vi "VESASignal_Run.vi"   [LabVIEW 2020]
uses:
  <vilib>/Platform/TimedLoop/XDataNode/timing_clust.ctl
  <vilib>/Platform/TimedLoop/XDataNode/nitl_modes.ctl
  <vilib>/Platform/TimedLoop/XDataNode/wakeup.ctl
  <vilib>/rvi/Emulation/niFpgaSctlEmulationGetInTimedLoop.vi
  <vilib>/rvi/Emulation/niFpgaEmulationReportErrorSimple.vi
  <vilib>/rvi/Emulation/niFpgaGetClockAttributes.vi
  <vilib>/rvi/Emulation/niFpgaCriticalErrorInLSC.vi
  <vilib>/rvi/Memory/Memory_Emulation/nirvimemoryFastEmulation.vi
  <vilib>/rvi/Memory/Memory_Emulation/nirvimemoryEmulation.vi
  <vilib>/rvi/Emulation/niFpgaEmulationIsFPGAContextNoSignature.vi
  <vilib>/rvi/DataTransferAndStorage/Container/Common/niFpgaContainerGetUniqueNameForEmu.vi
  <vilib>/rvi/Emulation/niFpgaProcessEmulError.vi
  <vilib>/rvi/errors/nirviReportUnexpectedCaseInternalError (U32).vi
  <vilib>/rvi/eio/common/nirviEmuTemplateMethod_errors.vi
  <vilib>/Platform/TimedLoop/XDataNode/XDataNode.xnode
  <vilib>/rvi/DataTransferAndStorage/Container/XNode/niFpgaContainer.xnode
  <vilib>/eio/EIONode/EIONode.xnode
  <vilib>/Platform/TimedLoop/XDataNode/XDNodeRunTimeDep.lvlib
types:
  T1 = typedef "XDNodeRunTimeDep.lvlib/timing_clust.ctl" = cluster{"Expected End [f-1]":u64, "Actual End [f-1]":u64, "Finished Late? [f-1]":bool, "Expected End [i-1]":u64, "Actual End [i-1]":u64, "Finished Late? [i-1]":bool, "Expected Start [i]":u64, "Actual Start [i]":u64, "Expected Start [f]":u64, "Actual Start [f]":u64, "Source Name":string, "Structure Name":string, "Period":i64, "Deadline":i64, "Offset":i64, "Start":i64, "Priority":i32, "Timeout":i32, "Mode":T2, "Wakeup Reason":T3, "Error":errorcluster, "Source Type":string, "Secondary Source Type":string, "Global End Time":u64, "Global Start Time":u64, "Frame Duration":u64, "Iteration Duration":u64, "Assigned CPU":i32, "I/O Scan Engine Mode":u32}
  T2 = typedef "XDNodeRunTimeDep.lvlib/nitl_modes.ctl" = enum32{"No Change", "Process missed periods, maintain original phase", "Discard missed periods, maintain original phase", "Process missed periods, ignore original phase", "Discard missed periods, ignore original phase"}
  T3 = typedef "XDNodeRunTimeDep.lvlib/wakeup.ctl" = enum32{"Normal", "Aborted", "Asynchronous wakeup", "Timing source error", "Timed loop error", "Timeout"}
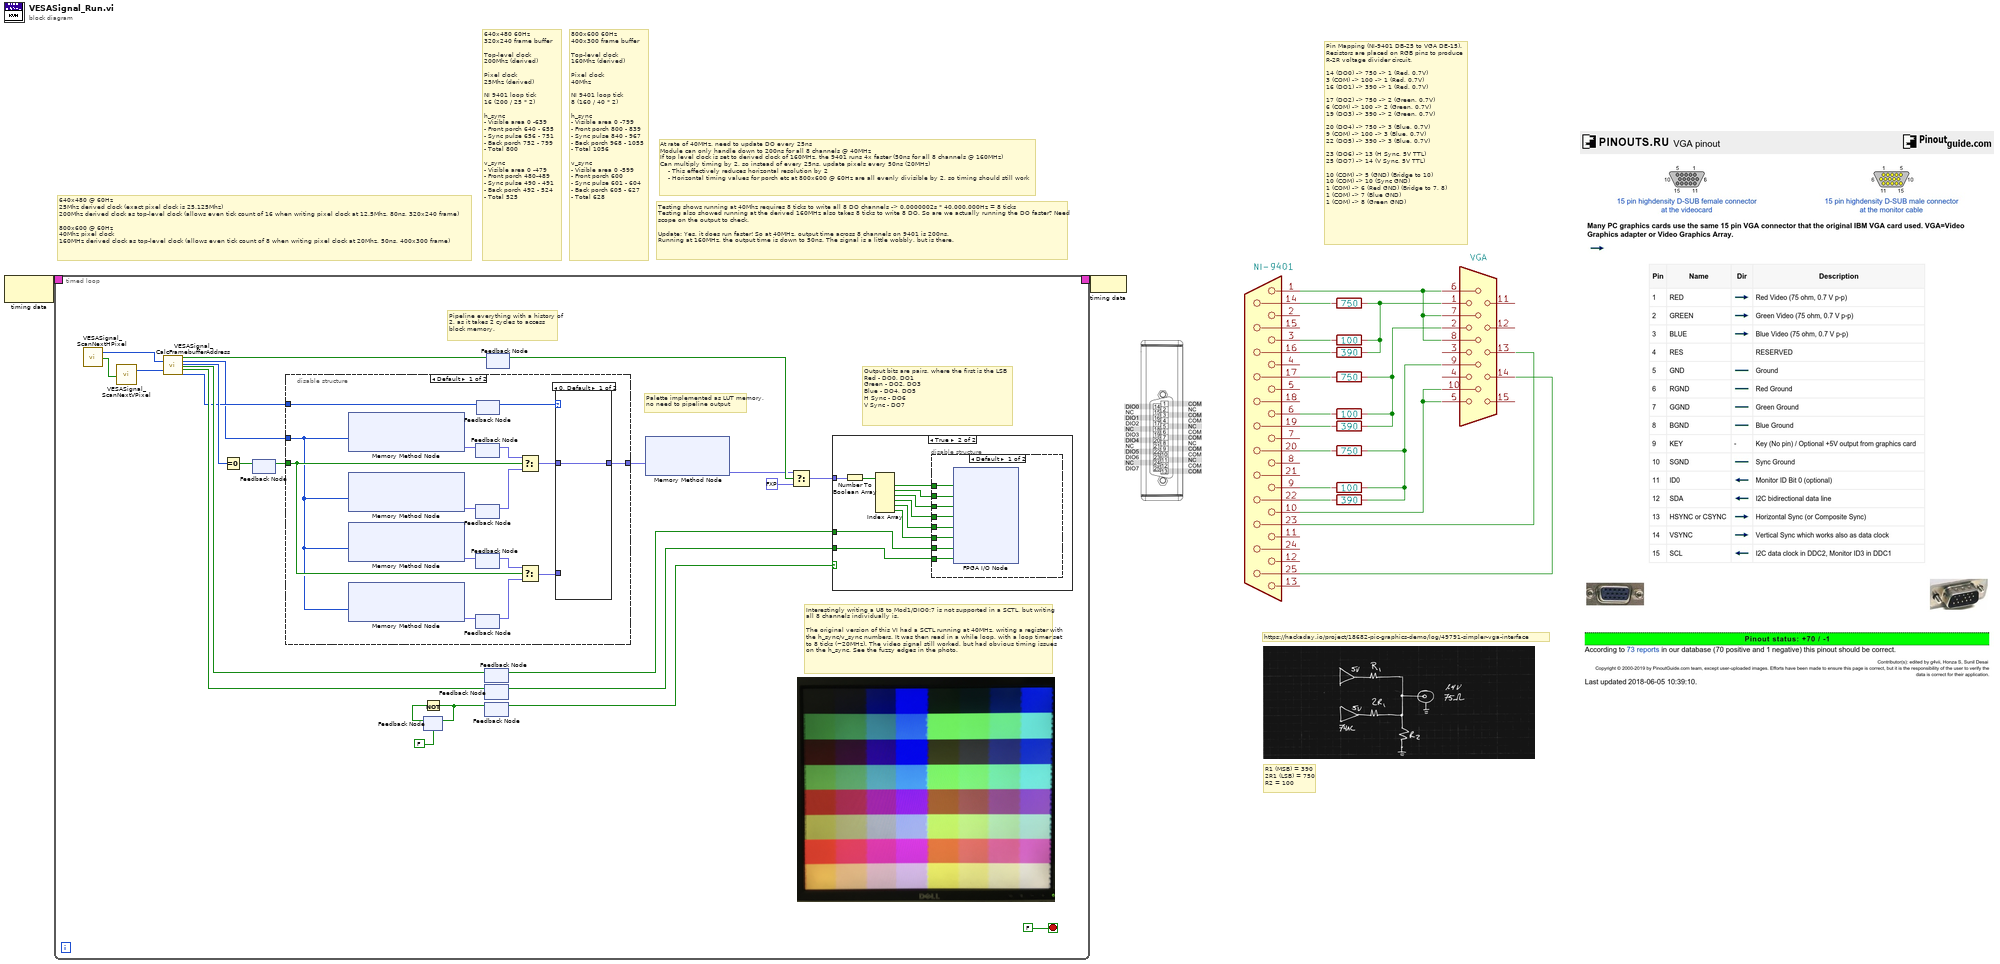
[diagram p0: block diagram]
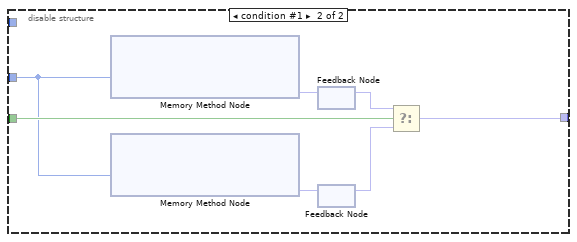
[diagram p3: hidden frame]
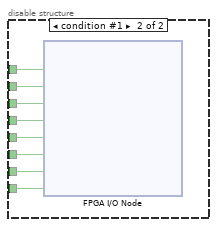
[diagram p5: hidden frame]
diagram:
  # "https://hackaday.io/project/18682-pic-graphics-demo/log/49791-simpler-vga-interface"
  # "R1 (MSB) = 390\n2R1 (LSB) = 750\nR2 = 100"
  # "Pin Mapping (NI-9401 DB-25 to VGA DE-15). Resistors are placed on RGB pins to produce R-2R voltage divider circuit.\n\n14 (DO0) -> 750 -> 1 (Red, 0.7V)\n3 (COM) -> 100 -> 1 (Red, 0.7V)\n16 (DO1) -> 390 -> 1 (Red, 0.7V)\n\n17 (DO2) -> 750 -> 2 (Green, 0.7V)\n6 (COM) -> 100 -> 2 (Green, 0.7V)\n19 (DO3) -> 390 -> 2 (Green, 0.7V)\n\n20 (DO4) -> 750 -> 3 (Blue, 0.7V)\n9 (COM) -> 100 -> 3 (Blue, 0.7V)\n22 (DO5) -> 390 -> 3 (Blue, 0.7V)\n\n23 (DO6) -> 13 (H Sync, 5V TTL)\n25 (DO7) -> 14 (V Sync, 5V TTL)\n\n10 (COM) -> 5 (GND) (Bridge to 10)\n10 (COM) -> 10 (Sync GND)\n1 (COM) -> 6 (Red GND) (Bridge to 7, 8)\n1 (COM) -> 7 (Blue GND)\n1 (COM) -> 8 (Green GND)"
  # "Testing shows running at 40Mhz requires 8 ticks to write all 8 DO channels -> 0.0000002s * 40,000,000Hz = 8 ticks \nTesting also showed running at the derived 160MHz also takes 8 ticks to write 8 DO. So are we actually running the DO faster? Need scope on the output to check.\n\nUpdate: Yes, it does run faster! So at 40MHz, output time across 8 channels on 9401 is 200ns.\nRunning at 160MHz, the output time is down to 50ns. The signal is a little wobbly, but is there."
  # "At rate of 40MHz, need to update DO every 25ns\nModule can only handle down to 200ns for all 8 channels @ 40MHz\nIf top level clock is set to derived clock of 160MHz, the 9401 runs 4x faster (50ns for all 8 channels @ 160MHz)\nCan multiply timing by 2, so instead of every 25ns, update pixels every 50ns (20MHz)\n    - This effectively reduces horizontal resolution by 2\n    - Horizontal timing values for porch etc at 800x600 @ 60Hz are all evenly divisible by 2, so timing should still work"
  # "800x600 60Hz\n400x300 frame buffer\n\nTop-level clock\n160Mhz (derived)\n\nPixel clock\n40Mhz\n\nNI 9401 loop tick\n8 (160 / 40 * 2)\n\nh_sync\n- Visible area 0 -799\n- Front porch 800 - 839\n- Sync pulse 840 - 967\n- Back porch 968 - 1055\n- Total 1056\n\nv_sync\n- Visible area 0 -599\n- Front porch 600\n- Sync pulse 601 - 604\n- Back porch 605 - 627\n- Total 628"
  # "640x480 60Hz\n320x240 frame buffer\n\nTop-level clock\n200Mhz (derived)\n\nPixel clock\n25Mhz (derived)\n\nNI 9401 loop tick\n16 (200 / 25 * 2)\n\nh_sync\n- Visible area 0 -639\n- Front porch 640 - 655\n- Sync pulse 656 - 751\n- Back porch 752 - 799\n- Total 800\n\nv_sync\n- Visible area 0 -479\n- Front porch 480-489\n- Sync pulse 490 - 491\n- Back porch 492 - 524\n- Total 525"
  # "640x480 @ 60Hz\n25Mhz derived clock (exact pixel clock is 25.125Mhz)\n200Mhz derived clock as top-level clock (allows even tick count of 16 when writing pixel clock at 12.5Mhz, 80ns, 320x240 frame)\n\n800x600 @ 60Hz\n40Mhz pixel clock\n160MHz derived clock as top-level clock (allows even tick count of 8 when writing pixel clock at 20Mhz, 50ns, 400x300 frame)"
  n1 = node-c288() -> (w2:T1)  [unwired: 1 in]
  n2 = timed-loop {
    timing: w2 -> [_]
    timing-out: [_] -> w1
    stop <- FALSE stop-if-true
    # "Interestingly writing a U8 to Mod1/DIO0:7 is not supported in a SCTL, but writing all 8 channels individually is.\n\nThe original version of this VI had a SCTL running at 40MHz, writing a register with the h_sync/v_sync numbers. It was then read in a while loop, with a loop timer set to 8 ticks (~20MHz). The video signal still worked, but had obvious timing issues on the h_sync. See the fuzzy edges in the photo."
    # "Output bits are pairs, where the first is the LSB\nRed - DO0, DO1\nGreen - DO2, DO3\nBlue - DO4, DO5\nH Sync - DO6\nV Sync - DO7"
    # "Pipeline everything with a history of 2, as it takes 2 cycles to access block memory."
    # "Palette implemented as LUT memory, no need to pipeline output"
    n3 = call "VESASignal_ScanNextHPixel.vi"() -> ("h_Pixel"=w23:i16, "Enable"=w22:bool)  [unwired: 18 in]
    n4 = call "VESASignal_ScanNextVPixel.vi"("Enable"=w22) -> ("v_Pixel"=w24:i16)  [unwired: 18 in]
    n5 = call "VESASignal_CalcFramebufferAddress.vi"("h_Pixel"=w23, "v_Pixel"=w24) -> ("draw_pixel"=w14:bool, "Address"=w3:u32, "buffer"=w13:u8, "h_sync"=w17:bool, "v_sync"=w16:bool, "Sub Buffer"=w5:u8)  [unwired: 12 in]
    n6 = Equal To 0?(x=w13) -> (x = 0?=w7:bool)
    n7 = feedback #1() -> (w6:bool)  [unwired: 1 in]
    n8 = feedback-in #1(w7) -> ()
    n9 = disable-structure shown="Default" {
      disable-tunnel: [w30 w43] -> w8
      disable-tunnel: w6 -> [w29 w45]
      disable-tunnel: w5 -> [w28 _]
      disable-tunnel: w3 -> [w26 w44]
      frame condition #0 (active) {
        n10 = xnode ("Memory Method Node")("Address"=w26) -> ("Data"=w32:fxp<+,6,6>)  [unwired: 1 in, 1 out]
        n11 = xnode ("Memory Method Node")("Address"=w26) -> ("Data"=w33:fxp<+,6,6>)  [unwired: 1 in, 1 out]
        n12 = xnode ("Memory Method Node")("Address"=w26) -> ("Data"=w40:fxp<+,6,6>)  [unwired: 1 in, 1 out]
        n13 = xnode ("Memory Method Node")("Address"=w26) -> ("Data"=w39:fxp<+,6,6>)  [unwired: 1 in, 1 out]
        n14 = feedback #2() -> (w34:fxp<+,6,6>)  [unwired: 1 in]
        n15 = feedback-in #2(w32) -> ()
        n16 = feedback #3() -> (w35:fxp<+,6,6>)  [unwired: 1 in]
        n17 = feedback-in #3(w33) -> ()
        n18 = feedback #4() -> (w38:fxp<+,6,6>)  [unwired: 1 in]
        n19 = feedback-in #4(w40) -> ()
        n20 = feedback #5() -> (w37:fxp<+,6,6>)  [unwired: 1 in]
        n21 = feedback-in #5(w39) -> ()
        n22 = feedback #6() -> (w27:u8)  [unwired: 1 in]
        n23 = feedback-in #6(w28) -> ()
        n24 = Select(t=w34, s=w29, f=w35) -> (s? t:f=w31:fxp<+,6,6>)
        n25 = Select(t=w38, s=w29, f=w37) -> (s? t:f=w36:fxp<+,6,6>)
        n26 = case shown="0, Default" w27 {
          tunnel: w36 -> [_ w42]
          tunnel: w31 -> [w41 _]
          tunnel: [w41 w42] -> w30
          frame 0, Default {
          }
          frame 1 {
          }
        }
      }
      frame condition #1 {
        n27 = xnode ("Memory Method Node")("Address"=w44) -> ("Data"=w46:fxp<+,6,6>)  [unwired: 1 in, 1 out]
        n28 = xnode ("Memory Method Node")("Address"=w44) -> ("Data"=w47:fxp<+,6,6>)  [unwired: 1 in, 1 out]
        n29 = feedback #7() -> (w48:fxp<+,6,6>)  [unwired: 1 in]
        n30 = feedback-in #7(w46) -> ()
        n31 = feedback #8() -> (w49:fxp<+,6,6>)  [unwired: 1 in]
        n32 = feedback-in #8(w47) -> ()
        n33 = Select(t=w48, s=w45, f=w49) -> (s? t:f=w43:fxp<+,6,6>)
      }
    }
    n34 = feedback #9(FALSE) -> (w20:bool)
    n35 = Not(x=w20) -> (.not. x?=w19:bool)
    n36 = feedback-in #9(w19) -> ()
    n37 = feedback #10() -> (w11:bool)  [unwired: 1 in]
    n38 = feedback-in #10(w17) -> ()
    n39 = feedback #11() -> (w10:bool)  [unwired: 1 in]
    n40 = feedback-in #11(w16) -> ()
    n41 = feedback #12() -> (w9:bool)  [unwired: 1 in]
    n42 = feedback-in #12(w19) -> ()
    n43 = feedback #13() -> (w12:bool)  [unwired: 1 in]
    n44 = feedback-in #13(w14) -> ()
    n45 = xnode ("Memory Method Node")("Address"=w8) -> ("Data"=w4:fxp<+,6,6>)  [unwired: 1 in, 1 out]
    n46 = Select(t=w4, s=w12, f=fxp<+,6,6> 0.0) -> (s? t:f=w15:fxp<+,6,6>)
    n47 = case shown="True" w9 {
      tunnel: w15 -> [_ w52]
      tunnel: w11 -> [_ w51]
      tunnel: w10 -> [_ w50]
      frame False {
      }
      frame True {
        n48 = Number To Boolean Array(number=w52) -> (Boolean array=w59:bool[])
        n49 = Index Array(array=w59) -> (element #1=w58:bool, element #2=w57:bool, element #3=w56:bool, element #4=w55:bool, element #5=w54:bool, element #6=w53:bool)  [unwired: 6 in]
        n50 = disable-structure shown="Default" {
          disable-tunnel: w58 -> [w67 w75]
          disable-tunnel: w57 -> [w66 w74]
          disable-tunnel: w56 -> [w65 w73]
          disable-tunnel: w55 -> [w64 w72]
          disable-tunnel: w54 -> [w63 w71]
          disable-tunnel: w53 -> [w62 w70]
          disable-tunnel: w51 -> [w61 w69]
          disable-tunnel: w50 -> [w60 w68]
          frame condition #0 (active) {
            n51 = xnode "FPGA I/O Node"("Mod1/DIO0"=w67, "Mod1/DIO1"=w66, "Mod1/DIO2"=w65, "Mod1/DIO3"=w64, "Mod1/DIO4"=w63, "Mod1/DIO5"=w62, "Mod1/DIO6"=w61, "Mod1/DIO7"=w60) -> ()  [unwired: 8 in, 8 out]
          }
          frame condition #1 {
            n52 = xnode "FPGA I/O Node"("ConnectorA/DIO0"=w75, "ConnectorA/DIO1"=w74, "ConnectorA/DIO2"=w73, "ConnectorA/DIO3"=w72, "ConnectorA/DIO4"=w71, "ConnectorA/DIO5"=w70, "ConnectorA/DIO6"=w69, "ConnectorA/DIO7"=w68) -> ()  [unwired: 8 in, 8 out]
          }
        }
      }
    }
  }
  n53 = node-c288(w1) -> ()
